vi "Write Time.vi"(8 "error in (no error)":errorcluster, 10 "Conversion Time":T1=1 items=["High Speed", "High Resolution"], 11 "9213 in":refnum<class "9212.lvclass">) -> (0 "error out":errorcluster, 3 "9213 out":refnum<class "9212.lvclass">)   [LabVIEW 2019, in "Modules.lvlib" / "9212.lvclass"]
uses:
  9212.lvclass
  Conversion Time.ctl
  9212.lvclass/9212.ctl
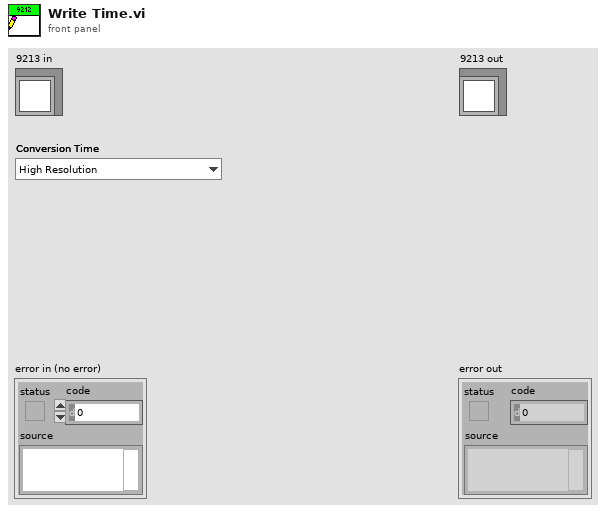
[diagram p1: front panel]
types:
  T1 = typedef "Modules.lvlib/9212.lvclass/Conversion Time.ctl" = u16
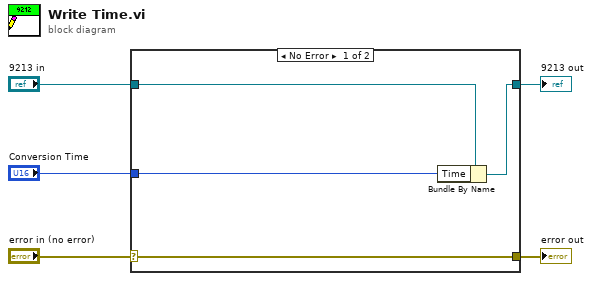
[diagram p0: block diagram]
diagram:
  n1 = case shown="No Error" "error in (no error)" {
    selector: "error in (no error)" -> [w9 w10]
    tunnel: [w9 w10] -> w4
    tunnel: [w7 w11] -> w2
    tunnel: "9213 in" -> [w8 w11]
    tunnel: "Conversion Time" -> [w6 _]
    frame No Error {
      n2 = Bundle By Name(cluster=w8, "Time"=w6) -> (w7:refnum<class "9212.lvclass">)
    }
    frame Error {
    }
  }
  "error out" <- w4
  "9213 out" <- w2
